vi "pressure control.vi"() -> ()   [LabVIEW 2019]
uses:
  <vilib>/measure/NI_MABase.lvlib
panel:
  out "Voltage input Error":waveform(dbl)(graph)
  out "contraction length":dbl(graph)
  out "Valve input voltage 2":waveform(dbl)(graph)
  out "linear pot 1":dbl(graph)
  out "linear pot":dbl format="%.4f"
  out "valve feeedback":dbl(graph)
  out "Valve input voltage":dbl(graph)
  out "Valve feedback (bar)":dbl format="%.4f"
  out "Valve input voltage":dbl format="%.4f"
  out "Voltage Gain":dbl
  out "Amplified Voltage":dbl format="%.4f"
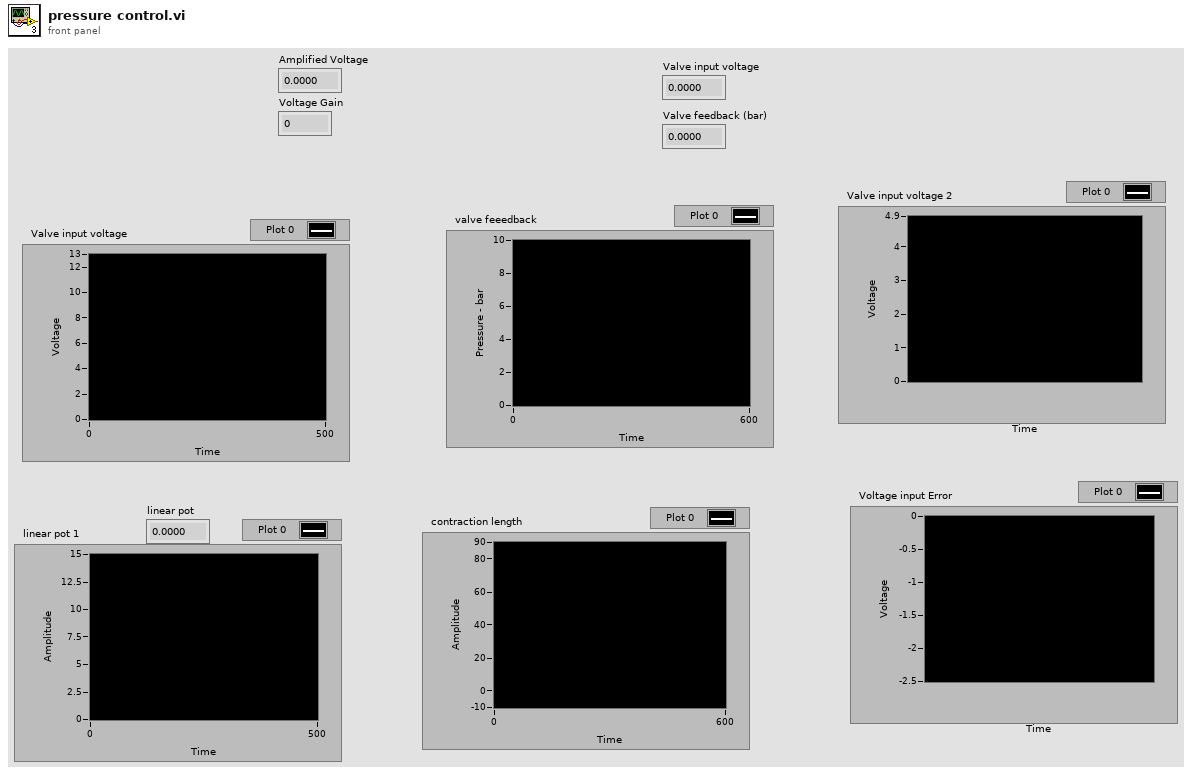
[diagram p1: front panel]
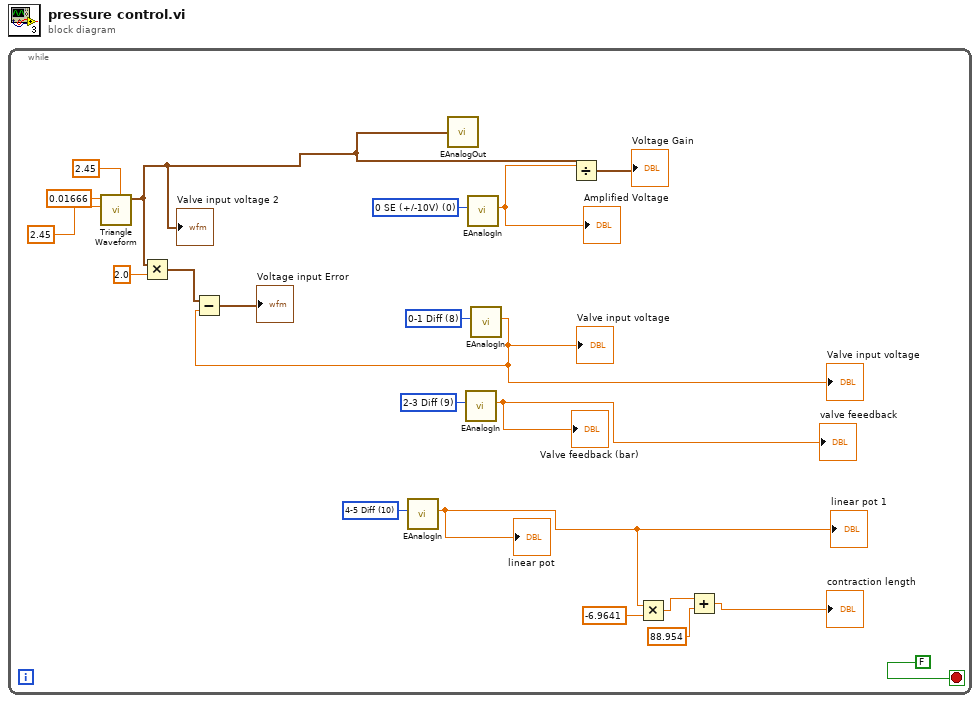
[diagram p0: block diagram]
diagram:
  n1 = while {
    stop <- FALSE stop-if-true
    w16 = u16 10 items=["0 SE (+/-10V)", "1 SE (+/-10V)", "2 SE (+/-10V)", "3 SE (+/-10V)", "4 SE (+/-10V)", "5 SE (+/-10V)", "6 SE (+/-10V)", "7 SE (+/-10V)", "0-1 Diff", "2-3 Diff", "4-5 Diff", "6-7 Diff"] ("Channel")
    w17 = u16 9 items=["0 SE (+/-10V)", "1 SE (+/-10V)", "2 SE (+/-10V)", "3 SE (+/-10V)", "4 SE (+/-10V)", "5 SE (+/-10V)", "6 SE (+/-10V)", "7 SE (+/-10V)", "0-1 Diff", "2-3 Diff", "4-5 Diff", "6-7 Diff"] ("Channel")
    w18 = u16 8 items=["0 SE (+/-10V)", "1 SE (+/-10V)", "2 SE (+/-10V)", "3 SE (+/-10V)", "4 SE (+/-10V)", "5 SE (+/-10V)", "6 SE (+/-10V)", "7 SE (+/-10V)", "0-1 Diff", "2-3 Diff", "4-5 Diff", "6-7 Diff"] ("Channel")
    w21 = u16 0 items=["0 SE (+/-10V)", "1 SE (+/-10V)", "2 SE (+/-10V)", "3 SE (+/-10V)", "4 SE (+/-10V)", "5 SE (+/-10V)", "6 SE (+/-10V)", "7 SE (+/-10V)", "0-1 Diff", "2-3 Diff", "4-5 Diff", "6-7 Diff"] ("Channel")
    n2 = call <vilib>:"Triangle Waveform.vi"("offset"=2.45, "amplitude"=2.45, "frequency"=0.01666) -> ("signal out"=w2:waveform(dbl))  [unwired: 7 in, 1 out]
    "Valve input voltage 2" <- w2
    n3 = Multiply(x=w2, y=2.0) -> (x*y=w4:waveform(dbl))
    n4 = call <vilib>:"EAnalogIn.vi"("Channel"=w16) -> ("Voltage"=w10:dbl)  [unwired: 6 in, 4 out]
    "linear pot" <- w10
    "linear pot 1" <- w10
    n5 = call <vilib>:"EAnalogOut.vi"("Analog Output 0 [volts]"=w2) -> ()  [unwired: 13 in, 2 out]
    n6 = call <vilib>:"EAnalogIn.vi"("Channel"=w17) -> ("Voltage"=→"Valve feedback (bar)" →"valve feeedback":dbl)  [unwired: 6 in, 4 out]
    n7 = call <vilib>:"EAnalogIn.vi"("Channel"=w21) -> ("Voltage"=w19:dbl)  [unwired: 6 in, 4 out]
    "Amplified Voltage" <- w19
    n8 = call <vilib>:"EAnalogIn.vi"("Channel"=w18) -> ("Voltage"=w3:dbl)  [unwired: 6 in, 4 out]
    "Valve input voltage" <- w3
    "Valve input voltage" <- w3
    n9 = Subtract(x=w4, y=w3) -> (x-y=→"Voltage input Error":waveform(dbl))
    n10 = Divide(x=w19, y=w2) -> (x/y=→"Voltage Gain":waveform(dbl))
    n11 = Multiply(x=w10, y=-6.9641) -> (x*y=w8:dbl)
    n12 = Add(x=w8, y=88.954) -> (x+y=→"contraction length":dbl)
  }
